vi "Timer and LED.vi"(9 "lines":tag, 10 "Stop":bool, 11 "Temperature":dbl) -> (2 "Tea Ready":bool, 3 "Elapsed Time (s)":dbl)   [LabVIEW 2022 SP3]
panel:
  in  "Threshold Temp":dbl
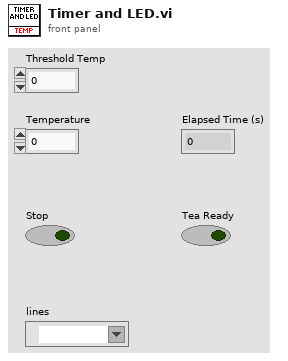
[diagram p1: front panel]
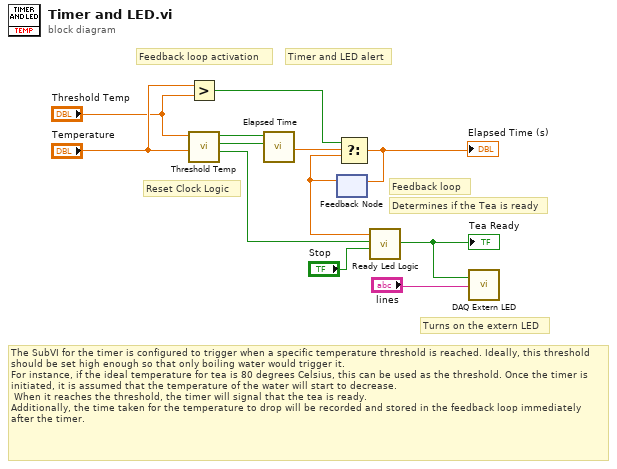
[diagram p0: block diagram]
diagram:
  # "Determines if the Tea is ready"
  # "Reset Clock Logic"
  # "Feedback loop activation"
  # "Timer and LED alert"
  # "Turns on the extern LED"
  # "The SubVI for the timer is configured to trigger when a specific temperature threshold is reached. Ideally, this threshold should be set high enough so that only boiling water would trigger it.\nFor instance, if the ideal temperature for tea is 80 degrees Celsius, this can be used as the threshold. Once the timer is initiated, it is assumed that the temperature of the water will start to decrease.\n When it reaches the threshold, the timer will signal that the tea is ready. \nAdditionally, the time taken for the temperature to drop will be recorded and stored in the feedback loop immediately after the timer."
  # "Feedback loop"
  n1 = Greater?(x="Temperature", y="Threshold Temp") -> (0:w7:bool)
  n2 = call "Threshold Temp.vi"("Temperature"="Temperature", "Temp Threshold"="Threshold Temp") -> ("Threshold Temp"=w9:bool, "Auto Reset"=w5:bool, "Reset"=w4:bool)  [unwired: 7 in]
  n3 = call "Elapsed Time"("Reset"=w4, "Auto Reset"=w5) -> ("Elapsed Time (s)"=w6:dbl)  [unwired: 10 in, 7 out]
  n4 = feedback #1() -> (w10:dbl)  [unwired: 1 in]
  n5 = Select(t=w6, s=w7, f=w10) -> (s? t:f=w8:dbl)
  "Elapsed Time (s)" <- w8
  n6 = feedback-in #1(w8) -> ()
  n7 = call "Ready Led Logic.vi"("Stop"="Stop", "Threshold Temp"=w9, "Elapsed Time (s)"=w10) -> ("Tea Ready"=w1:bool)  [unwired: 8 in]
  "Tea Ready" <- w1
  n8 = call "DAQ Extern LED.vi"("Tea Ready"=w1, "lines"="lines") -> ()  [unwired: 10 in]
